vi "write_spectrum_tdms.vi"(7 "timestamp":dbl format="%#_13g", 8 "error in (no error)":errorcluster, 9 "file path":path, 10 "SpectrumArray":dbl[](array[numeric]), 11 "WavelengthArray":dbl[](array[numeric])) -> (0 "error out":errorcluster, 1 "file path out":path)   [LabVIEW 2020, in "Thorlabs CCS175 Spectrometer.lvclass"]
uses:
  Thorlabs CCS175 Spectrometer.lvclass
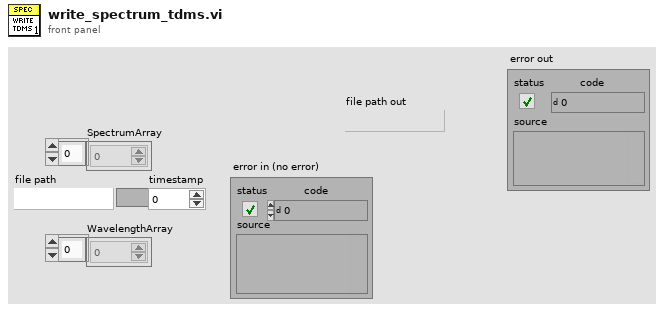
[diagram p1: front panel]
types:
  T1 = enum16{"open", "open or create", "create or replace", "create", "open (read-only)"}
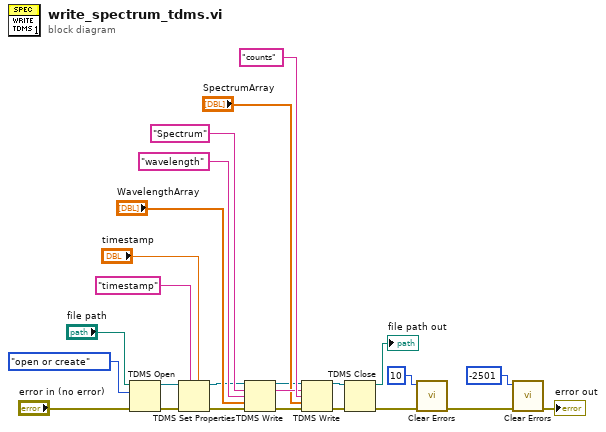
[diagram p0: block diagram]
diagram:
  n1 = TDMS Open(8:"error in (no error)", 10:T1."open or create" ("operation"), 11:"file path") -> (0:w11:errorcluster, 3:w12:refnum<k34>)  [unwired: 4 in]
  n2 = TDMS Set Properties(5:"timestamp", 7:"timestamp", 8:w11, 11:w12) -> (0:w16:errorcluster, 3:w14:refnum<k34>)  [unwired: 2 in, 2 out]
  n3 = TDMS Write(0:w14, 5:"Spectrum" ("group name in (Untitled)"), 7:"wavelength" ("channel name"), 9:"WavelengthArray", 11:w16) -> (4:w15:refnum<k34>, 6:w21:string, 15:w17:errorcluster)  [unwired: 1 in, 1 out]
  n4 = TDMS Write(0:w15, 5:w21, 7:"counts" ("channel name"), 9:"SpectrumArray", 11:w17) -> (4:w23:refnum<k34>, 15:w24:errorcluster)  [unwired: 1 in, 2 out]
  n5 = TDMS Close(8:w24, 11:w23) -> (0:w10:errorcluster, 3:→"file path out":path)
  n6 = call <vilib>:"Clear Errors.vi"("error in (no error)"=w10, "specific error code to clear (0: all)"=10) -> ("error out"=w8:errorcluster)  [unwired: 4 in, 1 out]
  n7 = call <vilib>:"Clear Errors.vi"("error in (no error)"=w8, "specific error code to clear (0: all)"=-2501) -> ("error out"=→"error out":errorcluster)  [unwired: 4 in, 1 out]
